vi "sweep_Gadi.vi"(0 "Stop  Frequency (1000.0 Hz)":dbl=1000.0 format="%#.6g", 1 "Start Frequency (100.0 Hz)":dbl=100.0 format="%#.6g", 2 "VISA resource name in":refnum<visa-resource-name>="K-33511B-03409", 3 "error in (no error)":errorcluster, 4 "Sweep Time (1.00 s)":dbl=1.0 format="%#.6g") -> ()   [LabVIEW 2016]
uses:
  <instrlib>/Agilent 33XXX Series/Agilent 33XXX Series.lvlib
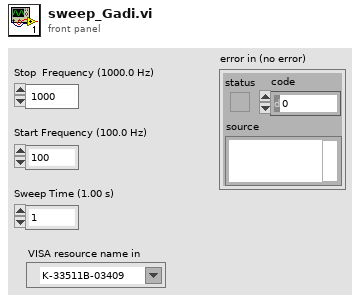
[diagram p1: front panel]
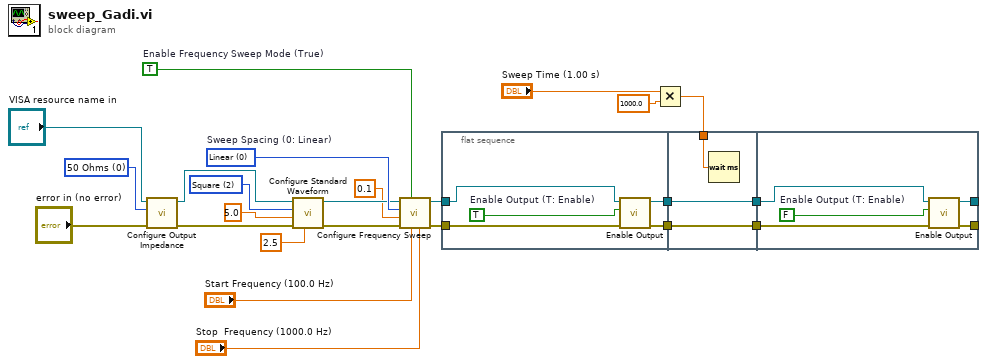
[diagram p0: block diagram]
diagram:
  w3 = u16 0 items=["50 Ohms", "High Impedance", "User Defined"] ("Impedance (0: 50 Ohms)")
  w13 = u16 2 items=["DC", "Sine", "Square", "Triangle", "Ramp", "Pulse", "Noise", "Sinc", "Negative Ramp", "Exponential Rise", "Exponential Fall", "Cardiac"] ("Waveform Function (1: Sine)")
  w16 = u16 0 items=["Linear", "Logarithmic"]  # Sweep Spacing (0: Linear)
  w10 = TRUE  # Enable Frequency Sweep Mode (True)
  n1 = call <instrlib>:"Configure Output Impedance.vi"("error in (no error)"="error in (no error)", "Impedance (0: 50 Ohms)"=w3, "VISA resource name"="VISA resource name in") -> ("error out"=w4:errorcluster, "VISA resource name out"=w5:refnum<visa-resource-name>)  [unwired: 7 in]
  n2 = call <instrlib>:"Configure Standard Waveform.vi"("DC Offset (0.00 V)"=2.5, "error in (no error)"=w4, "Amplitude (1)"=5.0 ("Amplitude (1 Vpp)"), "Waveform Function (1: Sine)"=w13, "VISA resource name"=w5) -> ("error out"=w7:errorcluster, "VISA resource name out"=w8:refnum<visa-resource-name>)  [unwired: 5 in]
  n3 = call <instrlib>:"Configure Frequency Sweep.vi"("Stop  Frequency (1000.0 Hz)"="Stop  Frequency (1000.0 Hz)", "Start Frequency (100.0 Hz)"="Start Frequency (100.0 Hz)", "Enable Frequency Sweep Mode (T: Enable)"=w10, "error in (no error)"=w7, "Sweep Time (1.00 s)"=0.1, "Sweep Spacing (0: Linear)"=w16, "VISA resource name"=w8) -> ("error out"=w15:errorcluster, "VISA resource name out"=w14:refnum<visa-resource-name>)  [unwired: 3 in]
  n4 = flat-sequence {
    tunnel: w14 -> [w29]
    tunnel: w15 -> [w28]
    tunnel: [w26] -> w24
    tunnel: [w25] -> w23
    tunnel: w20 -> [w32]
    tunnel: [w31] -> w22
    tunnel: w24 -> [w31]
    tunnel: [w30] -> w21
    tunnel: w23 -> [w30]
    tunnel: w22 -> [w36]
    tunnel: w21 -> [w35]
    tunnel: [w34] -> _
    tunnel: [w33] -> _
    frame #0 {
      w27 = TRUE  # Enable Output (T: Enable)
      n5 = call <instrlib>:"Enable Output.vi"("error in (no error)"=w28, "Enable Output  (T: Enable)"=w27, "VISA resource name"=w29) -> ("error out"=w25:errorcluster, "VISA resource name out"=w26:refnum<visa-resource-name>)  [unwired: 7 in]
    }
    frame #1 {
      n6 = Wait (ms)(milliseconds to wait=w32) -> ()  [unwired: 1 out]
    }
    frame #2 {
      w37 = FALSE  # Enable Output (T: Enable)
      n7 = call <instrlib>:"Enable Output.vi"("error in (no error)"=w35, "Enable Output  (T: Enable)"=w37, "VISA resource name"=w36) -> ("error out"=w33:errorcluster, "VISA resource name out"=w34:refnum<visa-resource-name>)  [unwired: 7 in]
    }
  }
  n8 = Multiply(x="Sweep Time (1.00 s)", y=1000.0) -> (x*y=w20:dbl)
